vi "GenerateDiploma.vi"(6 "Reprint":bool, 7 "printer name (default)":string="CutePDF Writer", 8 "error in (no error)":errorcluster, 9 "Path":path, 10 "Diplom":T1={"Name"="", "Swim Length"="", "With Aids"=TRUE, "Date"=timestamp(0 s since 1904-01-01), "Unit"=""}, 11 "Diploma In":T1[](array[typedef])) -> (0 "error out":errorcluster, 3 "Diploma Out":T1[](array[typedef]))   [LabVIEW 2018]
uses:
  TypeDef/Diploma.ctl
  <vilib>/Utility/miscctls.llb/LVPointTypeDef.ctl
panel:
  in  "Cancel Button":bool
  in  "Print Button":bool
  in  "Aids":bool
  in  "Længde":string
  in  "Navn":string
  # "Meter"
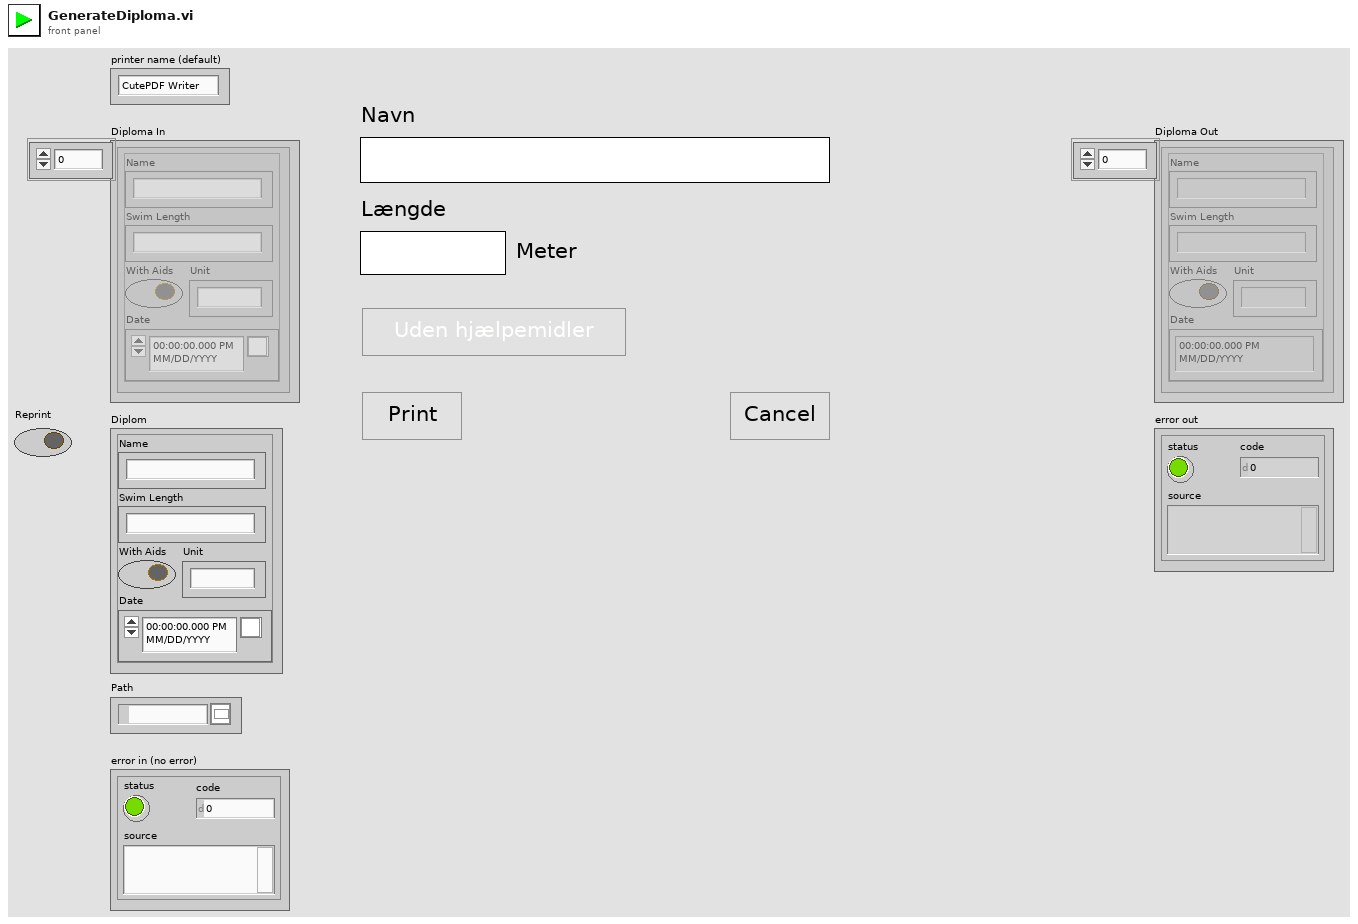
[diagram p1: front panel]
types:
  T1 = typedef "Diploma.ctl" = cluster{"Name":string, "Swim Length":string, "With Aids":bool, "Date":timestamp, "Unit":string}
  T2 = typedef "LVPointTypeDef.ctl" = cluster{"Horizontal":i16, "Vertical":i16}
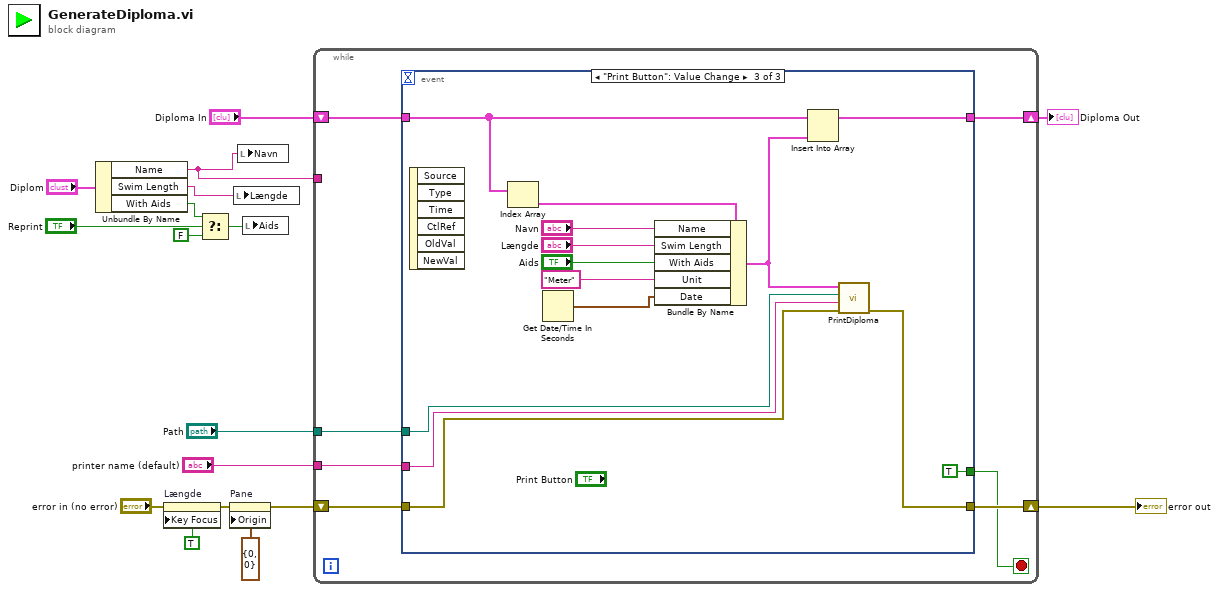
[diagram p0: block diagram]
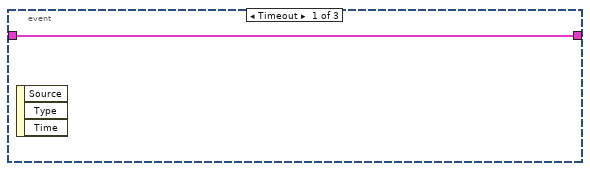
[diagram p2: hidden frame]
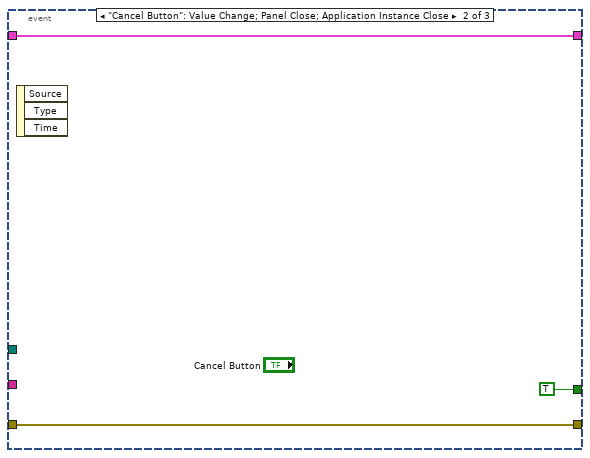
[diagram p3: hidden frame]
diagram:
  n1 = Unbundle By Name("Diplom") -> ("Name"=w8:string, "Swim Length"=w7:string, "With Aids"=w2:bool)
  n2 = property on="Længde" class="Str"(error in="error in (no error)", "Key Focus"=TRUE) -> (error out=w10:errorcluster)  [unwired: 1 in, 1 out]
  n3 = Select(t=w2, s="Reprint", f=FALSE) -> (s? t:f=w1:bool)
  n4 = property on="Pane" class="Pane"(error in=w10, "Origin"=T2 {"Horizontal"=0, "Vertical"=0}) -> (error out=w13:errorcluster)  [unwired: 1 in, 1 out]
  n5 = local write "Længde"(w7) -> ()
  n6 = local write "Navn"(w8) -> ()
  n7 = local write "Aids"(w1) -> ()
  n8 = while {
    shift-right: [w23] -> w16
    shift-left: "Diploma In" -> [w24]
    tunnel: "Path" -> [w20]
    shift-right: [w22] -> w6
    shift-left: w13 -> [w21]
    tunnel: w8 -> [_]
    tunnel: "printer name (default)" -> [w18]
    stop <- w19 stop-if-true
    n9 = event shown="[2] \"Print Button\": Value Change" {
      selector: _ -> [_ _ _]
      dyn-events: _ -> [_ _ _]
      timeout: _ -> [_ _ _]
      tunnel: w24 -> [w25 w28 w38]
      tunnel: [w25 w28 w37] -> w23
      tunnel: [_ w27 w36] -> w22
      tunnel: w21 -> [_ w27 w35]
      tunnel: w20 -> [_ _ w33]
      tunnel: [_ TRUE TRUE] -> w19
      tunnel: w18 -> [_ _ w29]
      event Timeout {
        n10 = event-data() -> ()  [unwired: 1 in, 3 out]
      }
      event "Cancel Button": Value Change; Panel Close; Application Instance Close {
        n11 = event-data() -> ()  [unwired: 1 in, 3 out]
      }
      event "Print Button": Value Change {
        n12 = event-data() -> ()  [unwired: 1 in, 6 out]
        n13 = Index Array(array=w38) -> (element=w42:T1)  [unwired: 1 in]
        n14 = Get Date/Time In Seconds() -> (seconds since 1Jan1904=w31:timestamp)
        n15 = Bundle By Name(cluster=w42, "Name"="Navn", "Swim Length"="Længde", "With Aids"="Aids", "Unit"="Meter", "Date"=w31) -> (w34:T1)
        n16 = Insert Into Array(array=w38, new element=w34) -> (w37:T1[])  [unwired: 1 in]
        n17 = call "PrintDiploma.vi"("error in (no error)"=w35, "printer name (default)"=w29, "Path"=w33, "Diploma"=w34) -> ("error out"=w36:errorcluster)  [unwired: 7 in]
      }
    }
  }
  "Diploma Out" <- w16
  "error out" <- w6
